vi "Error.vi"(8 "error in (no error)":errorcluster) -> ()   [LabVIEW 2013]
panel:
  out "Contour Plot":picture
  out "error out":errorcluster
  # "Whoops"
  # "We apologize; an error occured while initializing the demo\nprogram.  Please let us know so that we can investigate!\n\nYou can contact us at http://advancedplotting.com."
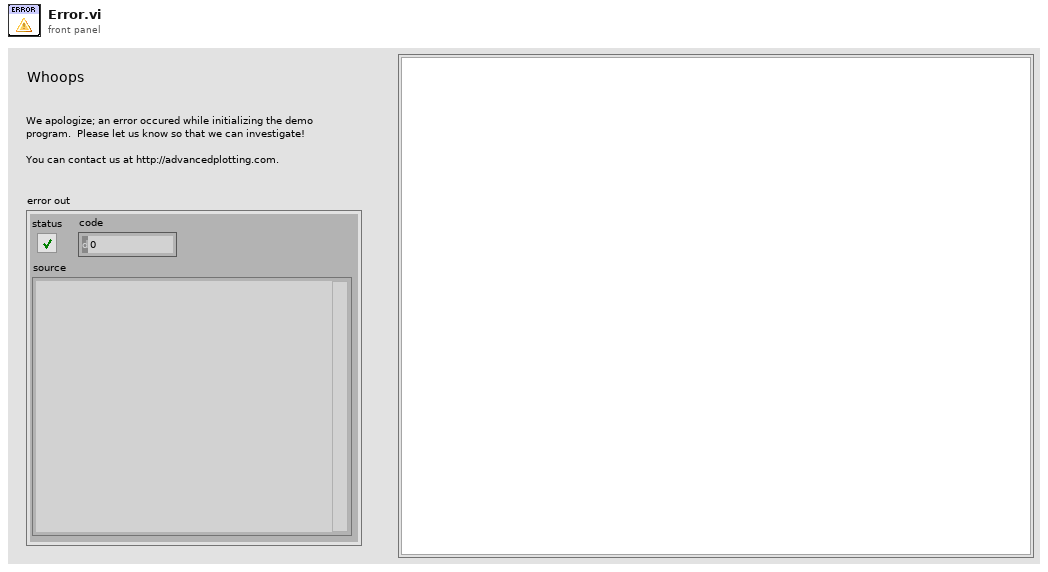
[diagram p1: front panel]
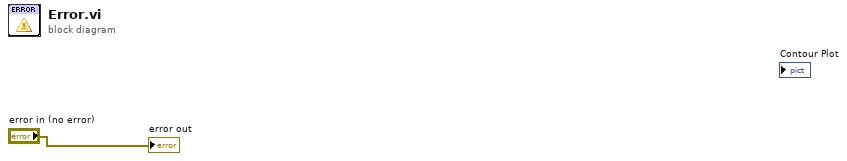
[diagram p0: block diagram]
diagram:
  "error out" <- "error in (no error)"
